vi "CAL-Compute Forward Response.vi"(0 "Y":dbl[](array[numeric]), 1 "Calibration file":path, 7 "Fs (Hz)":dbl) -> (3 "dB SPL":dbl, 4 "Yfilt":dbl[](array[numeric]), 6 "Freq (Hz)":dbl[](array[numeric]), 8 "Magnitude (dB)":dbl[](array[numeric]), 10 "Phase (degrees)":dbl[](array[numeric]))   [LabVIEW 2015]
uses:
  Utility VIs/Math VIs/LinSpace (x0-dx-npts).vi
  Utility VIs/Math VIs/FFT x(t) to dB,Degrees (1D).vi
  Utility VIs/Math VIs/Linear to dB (scalar).vi
  Utility VIs/Math VIs/Z to dB, degrees (1D).vi
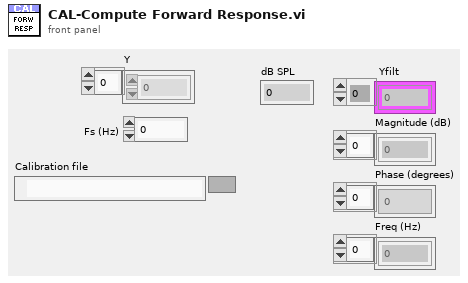
[diagram p1: front panel]
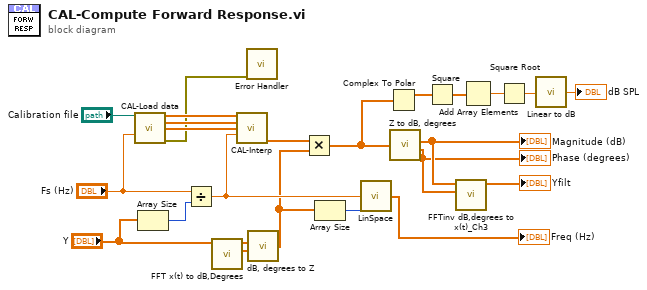
[diagram p0: block diagram]
diagram:
  n1 = call "CAL-Load data.vi"("user path"="Calibration file", "Desired Fs (Hz)"="Fs (Hz)") -> ("Frequency (Hz)"=w23:dbl[], "Mag"=w22:dbl[], "Phase"=w21:dbl[], "error out"=w14:errorcluster)  [unwired: 6 in, 4 out]
  n2 = Array Size(array="Y") -> (size(s)=w20:i32)
  n3 = Divide(x="Fs (Hz)", y=w20) -> (x/y=w10:dbl)
  n4 = call-poly "FFT x(t) to dB,Degrees.vi"("X"="Y") -> ("+Freq Phase of FFT (degrees)"=w17:dbl[], "+Freq. Mag of FFT (dB rms)"=w18:dbl[])  [unwired: 8 in, 1 out]
  n5 = call "CAL-Interp.vi"("Frequency (Hz)"=w23, "Magnitude (dB)"=w22, "Phase (degrees)"=w21, "df (Hz)"=w10) -> ("Interp z"=w16:cdb[])  [unwired: 8 in, 3 out]
  n6 = call "Error Handler.vi"("error in (no error)"=w14) -> ()  [unwired: 13 in, 2 out]
  n7 = call "dB, degrees to Z.vi"("Magnitude (dB)"=w18, "Phase (degrees)"=w17) -> ("Z"=w8:cdb[])  [unwired: 5 in]
  n8 = Multiply(x=w16, y=w8) -> (x*y=w6:cdb[])
  n9 = Array Size(array=w8) -> (size(s)=w9:i32)
  n10 = call-poly "LinSpace.vi"("npts"=w9, "dx"=w10) -> ("Array"=→"Freq (Hz)":dbl[])  [unwired: 2 in, 1 out]
  n11 = Complex To Polar(r * e^(i*theta)=w6) -> (r=w5:dbl[])  [unwired: 1 out]
  n12 = call-poly "Z to dB, degrees.vi"("Z"=w6) -> ("Magnitude (dB)"=w13:dbl[], "Phase (degrees)"=w12:dbl[])  [unwired: 5 in]
  "Magnitude (dB)" <- w13
  "Phase (degrees)" <- w12
  n13 = Square(x=w5) -> (x^2=w4:dbl[])
  n14 = call "FFTinv dB,degrees to x(t)_Ch3.vi"("+Freq Phase of FFT (degrees)"=w12, "+Freq. Mag of FFT (rms dB)"=w13) -> ("X(t)"=→"Yfilt":dbl[])  [unwired: 8 in, 1 out]
  n15 = Add Array Elements(numeric array=w4) -> (sum=w3:dbl)
  n16 = Square Root(x=w3) -> (sqrt(x)=w2:dbl)
  n17 = call-poly "Linear to dB.vi"("Linear"=w2) -> ("dB"=→"dB SPL":dbl)
